vi "Delete Float64Array DVR.vi"(8 "error in (no error)":errorcluster, 11 "Float64Array DVR in":refnum<data-value>) -> (0 "error out":errorcluster, 3 "Float64Array out":refnum<class "Float64Array.lvclass">)   [LabVIEW 2013, in "MDSplus.lvlib" / "Float64Array.lvclass"]
uses:
  <vilib>/MDSplus/Classes/Data_Class/Array_Class/Float64Array_Class/Float64Array.lvclass
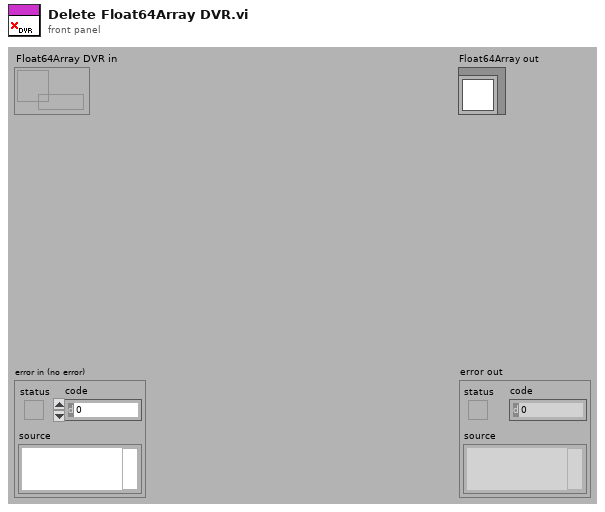
[diagram p1: front panel]
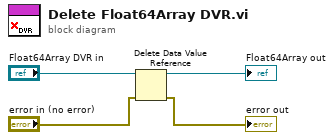
[diagram p0: block diagram]
diagram:
  n1 = Delete Data Value Reference(data value reference="Float64Array DVR in", error in="error in (no error)") -> (data value=→"Float64Array out":refnum<class "Float64Array.lvclass">, error out=→"error out":errorcluster)
